vi "XML File Path to VI File Path.vi"(11 "XML file path":path) -> (2 "keyword":string, 3 "VI file path":path)   [LabVIEW 2010, in "NI_SE_Front Panel Layout.lvlib"]
uses:
  NI_SE_Front Panel Layout.lvlib
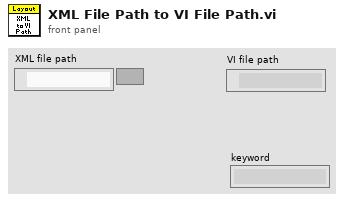
[diagram p1: front panel]
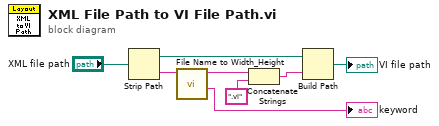
[diagram p0: block diagram]
diagram:
  n1 = Strip Path(path="XML file path") -> (stripped path=w4:path, name=w7:string)
  n2 = call "File Name to Width_Height.vi"("file name (with xml extension)"=w7) -> ("keyword"=→"keyword":string, "VI file name (no extension)"=w6:string)  [unwired: 7 in, 2 out]
  n3 = Concatenate Strings(w6, ".vi" ("string")) -> (w3:string)
  n4 = Build Path(base path=w4, name or relative path=w3) -> (appended path=→"VI file path":path)
